vi "Lab Panel V4.83.vi"() -> ()   [LabVIEW 2013] (continued)
                n1247 = Equal?(x=w2130, y=2) -> (x = y?=w2133:bool)
                n1248 = local read "DISP LAB03-2"() -> (w2135:T4)
                n1249 = Unbundle(w2135) -> ("STATUS"=w2136:string)  [unwired: 2 out]
                n1250 = Equal?(x=w2136, y="RUN") -> (x = y?=w2132:bool)
                n1251 = And(x=w2132, y=w2133) -> (x .and. y?=w2131:bool)
                n1252 = case shown="True" w2131 {
                  tunnel: w2135 -> [_ w2139]
                  tunnel: w2129 -> [_ w2142]
                  frame False {
                  }
                  frame True {
                    n1253 = local read "SET LAB03-2"() -> (w2141:T5)
                    n1254 = local read "TDMS LAB03-2"() -> (w2138:refnum<k34>)
                    n1255 = Unbundle(w2139) -> ("CYCLE"=w2143:dbl)  [unwired: 2 out]
                    n1256 = Unbundle(w2141) -> ("T-RISE mins"=w2140:dbl)  [unwired: 4 out]
                    n1257 = Greater Or Equal?(x=w2143, y=w2142) -> (x >= y?=w2144:bool)
                    n1258 = case shown="True" w2144 {
                      tunnel: w2140 -> [w2147 _]
                      tunnel: w2139 -> [w2146 _]
                      tunnel: w2138 -> [w2145 _]
                      frame True {
                        n1259 = stacked-sequence {
                          tunnel: w2147 -> [w2150 _]
                          tunnel: w2146 -> [_ w2155]
                          tunnel: w2145 -> [w2148 _]
                          frame #0 {
                            n1260 = Build Array("T-RISE") -> (w2152:string[])
                            n1261 = Build Array(w2150) -> (w2151:dbl[])
                            n1262 = TDMS Write(0:w2148, 5:"TEST PASS", 7:w2152, 9:w2151) -> (15:w2154:errorcluster)  [unwired: 2 in, 3 out]
                            n1263 = local write "data file error"(w2154) -> ()
                          }
                          frame #1 {
                            n1264 = Bundle(cluster=w2155, "STATUS"="T-RISE PASS") -> (w2157:T4)  [unwired: 2 in]
                            n1265 = local write "RESULT LAB03-2"(TRUE) -> ()
                            n1266 = local write "DISP LAB03-2"(w2157) -> ()
                          }
                        }
                      }
                      frame False {
                      }
                    }
                  }
                }
              }
              frame #6 {
                # "LAB04-1"
                n1267 = Equal?(x=w2160, y=2) -> (x = y?=w2163:bool)
                n1268 = local read "DISP LAB04-1"() -> (w2165:T4)
                n1269 = Unbundle(w2165) -> ("STATUS"=w2166:string)  [unwired: 2 out]
                n1270 = Equal?(x=w2166, y="RUN") -> (x = y?=w2162:bool)
                n1271 = And(x=w2162, y=w2163) -> (x .and. y?=w2161:bool)
                n1272 = case shown="True" w2161 {
                  tunnel: w2165 -> [_ w2169]
                  tunnel: w2159 -> [_ w2172]
                  frame False {
                  }
                  frame True {
                    n1273 = local read "SET LAB04-1"() -> (w2171:T5)
                    n1274 = local read "TDMS LAB04-1"() -> (w2168:refnum<k34>)
                    n1275 = Unbundle(w2169) -> ("CYCLE"=w2173:dbl)  [unwired: 2 out]
                    n1276 = Unbundle(w2171) -> ("T-RISE mins"=w2170:dbl)  [unwired: 4 out]
                    n1277 = Greater Or Equal?(x=w2173, y=w2172) -> (x >= y?=w2174:bool)
                    n1278 = case shown="True" w2174 {
                      tunnel: w2170 -> [w2177 _]
                      tunnel: w2169 -> [w2176 _]
                      tunnel: w2168 -> [w2175 _]
                      frame True {
                        n1279 = stacked-sequence {
                          tunnel: w2177 -> [w2180 _]
                          tunnel: w2176 -> [_ w2185]
                          tunnel: w2175 -> [w2178 _]
                          frame #0 {
                            n1280 = Build Array("T-RISE") -> (w2182:string[])
                            n1281 = Build Array(w2180) -> (w2181:dbl[])
                            n1282 = TDMS Write(0:w2178, 5:"TEST PASS", 7:w2182, 9:w2181) -> (15:w2184:errorcluster)  [unwired: 2 in, 3 out]
                            n1283 = local write "data file error"(w2184) -> ()
                          }
                          frame #1 {
                            n1284 = Bundle(cluster=w2185, "STATUS"="T-RISE PASS") -> (w2187:T4)  [unwired: 2 in]
                            n1285 = local write "RESULT LAB04-1"(TRUE) -> ()
                            n1286 = local write "DISP LAB04-1"(w2187) -> ()
                          }
                        }
                      }
                      frame False {
                      }
                    }
                  }
                }
              }
              frame #7 {
                # "LAB04-2"
                n1287 = Equal?(x=w2190, y=2) -> (x = y?=w2193:bool)
                n1288 = local read "DISP LAB04-2"() -> (w2195:T4)
                n1289 = Unbundle(w2195) -> ("STATUS"=w2196:string)  [unwired: 2 out]
                n1290 = Equal?(x=w2196, y="RUN") -> (x = y?=w2192:bool)
                n1291 = And(x=w2192, y=w2193) -> (x .and. y?=w2191:bool)
                n1292 = case shown="True" w2191 {
                  tunnel: w2195 -> [_ w2199]
                  tunnel: w2189 -> [_ w2202]
                  frame False {
                  }
                  frame True {
                    n1293 = local read "SET LAB04-2"() -> (w2201:T5)
                    n1294 = local read "TDMS LAB04-2"() -> (w2198:refnum<k34>)
                    n1295 = Unbundle(w2199) -> ("CYCLE"=w2203:dbl)  [unwired: 2 out]
                    n1296 = Unbundle(w2201) -> ("T-RISE mins"=w2200:dbl)  [unwired: 4 out]
                    n1297 = Greater Or Equal?(x=w2203, y=w2202) -> (x >= y?=w2204:bool)
                    n1298 = case shown="True" w2204 {
                      tunnel: w2200 -> [w2207 _]
                      tunnel: w2199 -> [w2206 _]
                      tunnel: w2198 -> [w2205 _]
                      frame True {
                        n1299 = stacked-sequence {
                          tunnel: w2207 -> [w2210 _]
                          tunnel: w2206 -> [_ w2215]
                          tunnel: w2205 -> [w2208 _]
                          frame #0 {
                            n1300 = Build Array("T-RISE") -> (w2212:string[])
                            n1301 = Build Array(w2210) -> (w2211:dbl[])
                            n1302 = TDMS Write(0:w2208, 5:"TEST PASS", 7:w2212, 9:w2211) -> (15:w2214:errorcluster)  [unwired: 2 in, 3 out]
                            n1303 = local write "data file error"(w2214) -> ()
                          }
                          frame #1 {
                            n1304 = Bundle(cluster=w2215, "STATUS"="T-RISE PASS") -> (w2217:T4)  [unwired: 2 in]
                            n1305 = local write "RESULT LAB04-2"(TRUE) -> ()
                            n1306 = local write "DISP LAB04-2"(w2217) -> ()
                          }
                        }
                      }
                      frame False {
                      }
                    }
                  }
                }
              }
              frame #8 {
                # "LAB05-1"
                n1307 = Equal?(x=w2220, y=2) -> (x = y?=w2223:bool)
                n1308 = local read "DISP LAB05-1"() -> (w2225:T4)
                n1309 = Unbundle(w2225) -> ("STATUS"=w2226:string)  [unwired: 2 out]
                n1310 = Equal?(x=w2226, y="RUN") -> (x = y?=w2222:bool)
                n1311 = And(x=w2222, y=w2223) -> (x .and. y?=w2221:bool)
                n1312 = case shown="True" w2221 {
                  tunnel: w2225 -> [_ w2229]
                  tunnel: w2219 -> [_ w2232]
                  frame False {
                  }
                  frame True {
                    n1313 = local read "SET LAB05-1"() -> (w2231:T5)
                    n1314 = local read "TDMS LAB05-1"() -> (w2228:refnum<k34>)
                    n1315 = Unbundle(w2229) -> ("CYCLE"=w2233:dbl)  [unwired: 2 out]
                    n1316 = Unbundle(w2231) -> ("T-RISE mins"=w2230:dbl)  [unwired: 4 out]
                    n1317 = Greater Or Equal?(x=w2233, y=w2232) -> (x >= y?=w2234:bool)
                    n1318 = case shown="True" w2234 {
                      tunnel: w2230 -> [w2237 _]
                      tunnel: w2229 -> [w2236 _]
                      tunnel: w2228 -> [w2235 _]
                      frame True {
                        n1319 = stacked-sequence {
                          tunnel: w2237 -> [w2240 _]
                          tunnel: w2236 -> [_ w2245]
                          tunnel: w2235 -> [w2238 _]
                          frame #0 {
                            n1320 = Build Array("T-RISE") -> (w2242:string[])
                            n1321 = Build Array(w2240) -> (w2241:dbl[])
                            n1322 = TDMS Write(0:w2238, 5:"TEST PASS", 7:w2242, 9:w2241) -> (15:w2244:errorcluster)  [unwired: 2 in, 3 out]
                            n1323 = local write "data file error"(w2244) -> ()
                          }
                          frame #1 {
                            n1324 = Bundle(cluster=w2245, "STATUS"="T-RISE PASS") -> (w2247:T4)  [unwired: 2 in]
                            n1325 = local write "RESULT LAB05-1"(TRUE) -> ()
                            n1326 = local write "DISP LAB05-1"(w2247) -> ()
                          }
                        }
                      }
                      frame False {
                      }
                    }
                  }
                }
              }
              frame #9 {
                # "LAB05-2"
                n1327 = Equal?(x=w2250, y=2) -> (x = y?=w2253:bool)
                n1328 = local read "DISP LAB05-2"() -> (w2255:T4)
                n1329 = Unbundle(w2255) -> ("STATUS"=w2256:string)  [unwired: 2 out]
                n1330 = Equal?(x=w2256, y="RUN") -> (x = y?=w2252:bool)
                n1331 = And(x=w2252, y=w2253) -> (x .and. y?=w2251:bool)
                n1332 = case shown="True" w2251 {
                  tunnel: w2255 -> [_ w2259]
                  tunnel: w2249 -> [_ w2262]
                  frame False {
                  }
                  frame True {
                    n1333 = local read "SET LAB05-2"() -> (w2261:T5)
                    n1334 = local read "TDMS LAB05-2"() -> (w2258:refnum<k34>)
                    n1335 = Unbundle(w2259) -> ("CYCLE"=w2263:dbl)  [unwired: 2 out]
                    n1336 = Unbundle(w2261) -> ("T-RISE mins"=w2260:dbl)  [unwired: 4 out]
                    n1337 = Greater Or Equal?(x=w2263, y=w2262) -> (x >= y?=w2264:bool)
                    n1338 = case shown="True" w2264 {
                      tunnel: w2260 -> [w2267 _]
                      tunnel: w2259 -> [w2266 _]
                      tunnel: w2258 -> [w2265 _]
                      frame True {
                        n1339 = stacked-sequence {
                          tunnel: w2267 -> [w2270 _]
                          tunnel: w2266 -> [_ w2275]
                          tunnel: w2265 -> [w2268 _]
                          frame #0 {
                            n1340 = Build Array("T-RISE") -> (w2272:string[])
                            n1341 = Build Array(w2270) -> (w2271:dbl[])
                            n1342 = TDMS Write(0:w2268, 5:"TEST PASS", 7:w2272, 9:w2271) -> (15:w2274:errorcluster)  [unwired: 2 in, 3 out]
                            n1343 = local write "data file error"(w2274) -> ()
                          }
                          frame #1 {
                            n1344 = Bundle(cluster=w2275, "STATUS"="T-RISE PASS") -> (w2277:T4)  [unwired: 2 in]
                            n1345 = local write "RESULT LAB05-2"(TRUE) -> ()
                            n1346 = local write "DISP LAB05-2"(w2277) -> ()
                          }
                        }
                      }
                      frame False {
                      }
                    }
                  }
                }
              }
            }
          }
          frame #6 {
            # "end test & close test files"
            n1347 = stacked-sequence {
              tunnel: w2288 -> [_ _ _ _ _ _ _ _ _ _]
              tunnel: w2289 -> [_ _ _ _ _ _ _ _ _ _]
              tunnel: w2287 -> [_ _ _ _ _ _ _ _ _ _]
              tunnel: w2286 -> [_ _ _ _ _ _ _ _ _ _]
              tunnel: w2285 -> [_ _ _ _ _ _ _ _ _ _]
              tunnel: w2284 -> [_ _ _ _ _ _ _ _ _ _]
              tunnel: w2283 -> [_ _ _ _ _ _ _ _ _ _]
              tunnel: w2282 -> [_ _ _ _ _ _ _ _ _ _]
              tunnel: w2281 -> [_ _ _ _ _ _ _ _ _ _]
              tunnel: w2280 -> [_ _ _ _ _ _ _ _ _ _]
              frame #0 {
                # "LAB01-1"
                n1348 = local read "DISP LAB01-1"() -> (w2293:T4)
                n1349 = local read "run lab01-1"() -> (w2290:bool)
                n1350 = local read "TDMS LAB01-1"() -> (w2291:refnum<k34>)
                n1351 = Unbundle(w2293) -> ("CYCLE"=w2294:dbl, "STATUS"=w2292:string)  [unwired: 1 out]
                n1352 = case shown="True" w2290 {
                  tunnel: w2294 -> [_ w2298]
                  tunnel: w2293 -> [_ w2297]
                  tunnel: w2292 -> [_ w2296]
                  tunnel: w2291 -> [_ w2295]
                  frame False {
                  }
                  frame True {
                    n1353 = Not Equal?(x=w2296, y="RUN") -> (x != y?=w2299:bool)
                    n1354 = Greater?(x=w2298, y=2.0) -> (0:w2301:bool)
                    n1355 = And(x=w2301, y=w2299) -> (x .and. y?=w2300:bool)
                    n1356 = case shown="True" w2300 {
                      tunnel: w2297 -> [_ w2305]
                      tunnel: w2295 -> [_ w2304]
                      frame False {
                      }
                      frame True {
                        n1357 = stacked-sequence {
                          tunnel: w2305 -> [w2309 _ _]
                          tunnel: w2304 -> [_ w2311 _]
                          frame #0 {
                            w2306 = FALSE
                            n1358 = local write "mail control"("END") -> ()
                            n1359 = Bundle(cluster=w2309) -> (w2308:T4)  [unwired: 3 in]
                            n1360 = local write "DISP LAB01-1"(w2308) -> ()
                            n1361 = local write "O/I  LAB01-1"(w2306) -> ()
                            n1362 = local write "run lab01-1"(w2306) -> ()
                            n1363 = local write "RUN LAB01-1"(w2306) -> ()
                          }
                          frame #1 {
                            n1364 = TDMS Close(11:w2311) -> (0:w2310:errorcluster)  [unwired: 1 in, 1 out]
                            n1365 = local write "data file error"(w2310) -> ()
                          }
                          frame #2 {
                            n1366 = stacked-sequence {
                              tunnel: "LAB01-1" -> [w2314 w2316]
                              frame #0 {
                                n1367 = call "sub vi - defrag tdms v1.vi"("panel id"=w2314) -> ("error out"=w2313:errorcluster)  [unwired: 10 in]
                                n1368 = local write "data file error"(w2313) -> ()
                              }
                              frame #1 {
                                n1369 = call "Save data file to network drive v1.vi"("panel id"=w2316) -> ("network file save error"=w2315:errorcluster)  [unwired: 9 in, 1 out]
                                n1370 = local write "data file error"(w2315) -> ()
                              }
                            }
                          }
                        }
                      }
                    }
                  }
                }
              }
              frame #1 {
                # "LAB01-2"
                n1371 = local read "run lab01-2"() -> (w2317:bool)
                n1372 = case shown="True" w2317 {
                  frame False {
                  }
                  frame True {
                    n1373 = local read "DISP LAB01-2"() -> (w2324:T4)
                    n1374 = local read "TDMS LAB01-2"() -> (w2323:refnum<k34>)
                    n1375 = Unbundle(w2324) -> ("CYCLE"=w2320:dbl, "STATUS"=w2325:string)  [unwired: 1 out]
                    n1376 = Not Equal?(x=w2325, y="RUN") -> (x != y?=w2319:bool)
                    n1377 = Greater?(x=w2320, y=2.0) -> (0:w2321:bool)
                    n1378 = And(x=w2321, y=w2319) -> (x .and. y?=w2318:bool)
                    n1379 = case shown="True" w2318 {
                      tunnel: w2324 -> [_ w2328]
                      tunnel: w2323 -> [_ w2327]
                      frame False {
                      }
                      frame True {
                        n1380 = stacked-sequence {
                          tunnel: w2328 -> [w2331 _ _]
                          tunnel: w2327 -> [_ w2333 _]
                          frame #0 {
                            w2329 = FALSE
                            n1381 = local write "mail control"("END") -> ()
                            n1382 = Bundle(cluster=w2331) -> (w2332:T4)  [unwired: 3 in]
                            n1383 = local write "RUN LAB01-2"(w2329) -> ()
                            n1384 = local write "run lab01-2"(w2329) -> ()
                            n1385 = local write "O/I  LAB01-2"(w2329) -> ()
                            n1386 = local write "DISP LAB01-2"(w2332) -> ()
                          }
                          frame #1 {
                            n1387 = TDMS Close(11:w2333) -> (0:w2334:errorcluster)  [unwired: 1 in, 1 out]
                            n1388 = local write "data file error"(w2334) -> ()
                          }
                          frame #2 {
                            n1389 = stacked-sequence {
                              tunnel: "LAB01-2" -> [w2337 w2339]
                              frame #0 {
                                n1390 = call "sub vi - defrag tdms v1.vi"("panel id"=w2337) -> ("error out"=w2336:errorcluster)  [unwired: 10 in]
                                n1391 = local write "data file error"(w2336) -> ()
                              }
                              frame #1 {
                                n1392 = call "Save data file to network drive v1.vi"("panel id"=w2339) -> ("network file save error"=w2338:errorcluster)  [unwired: 9 in, 1 out]
                                n1393 = local write "data file error"(w2338) -> ()
                              }
                            }
                          }
                        }
                      }
                    }
                  }
                }
              }
              frame #2 {
                # "LAB02-1"
                n1394 = local read "run lab02-1"() -> (w2340:bool)
                n1395 = case shown="True" w2340 {
                  frame False {
                  }
                  frame True {
                    n1396 = local read "DISP LAB02-1"() -> (w2347:T4)
                    n1397 = Unbundle(w2347) -> ("CYCLE"=w2343:dbl, "STATUS"=w2348:string)  [unwired: 1 out]
                    n1398 = local read "TDMS LAB02-1"() -> (w2346:refnum<k34>)
                    n1399 = Not Equal?(x=w2348, y="RUN") -> (x != y?=w2342:bool)
                    n1400 = Greater?(x=w2343, y=2.0) -> (0:w2344:bool)
                    n1401 = And(x=w2344, y=w2342) -> (x .and. y?=w2341:bool)
                    n1402 = case shown="True" w2341 {
                      tunnel: w2347 -> [_ w2351]
                      tunnel: w2346 -> [_ w2350]
                      frame False {
                      }
                      frame True {
                        n1403 = stacked-sequence {
                          tunnel: w2351 -> [w2354 _ _]
                          tunnel: w2350 -> [_ w2356 _]
                          frame #0 {
                            w2352 = FALSE
                            n1404 = local write "mail control"("END") -> ()
                            n1405 = Bundle(cluster=w2354) -> (w2355:T4)  [unwired: 3 in]
                            n1406 = local write "O/I  LAB02-1"(w2352) -> ()
                            n1407 = local write "RUN LAB02-1"(w2352) -> ()
                            n1408 = local write "run lab02-1"(w2352) -> ()
                            n1409 = local write "DISP LAB02-1"(w2355) -> ()
                          }
                          frame #1 {
                            n1410 = TDMS Close(11:w2356) -> (0:w2357:errorcluster)  [unwired: 1 in, 1 out]
                            n1411 = local write "data file error"(w2357) -> ()
                          }
                          frame #2 {
                            n1412 = stacked-sequence {
                              tunnel: "LAB02-1" -> [w2360 w2362]
                              frame #0 {
                                n1413 = call "sub vi - defrag tdms v1.vi"("panel id"=w2360) -> ("error out"=w2359:errorcluster)  [unwired: 10 in]
                                n1414 = local write "data file error"(w2359) -> ()
                              }
                              frame #1 {
                                n1415 = call "Save data file to network drive v1.vi"("panel id"=w2362) -> ("network file save error"=w2361:errorcluster)  [unwired: 9 in, 1 out]
                                n1416 = local write "data file error"(w2361) -> ()
                              }
                            }
                          }
                        }
                      }
                    }
                  }
                }
              }
              frame #3 {
                # "LAB02-2"
                n1417 = local read "run lab02-2"() -> (w2363:bool)
                n1418 = case shown="True" w2363 {
                  frame False {
                  }
                  frame True {
                    n1419 = local read "DISP LAB02-2"() -> (w2370:T4)
                    n1420 = local read "TDMS LAB02-2"() -> (w2369:refnum<k34>)
                    n1421 = Unbundle(w2370) -> ("CYCLE"=w2366:dbl, "STATUS"=w2371:string)  [unwired: 1 out]
                    n1422 = Not Equal?(x=w2371, y="RUN") -> (x != y?=w2365:bool)
                    n1423 = Greater?(x=w2366, y=2.0) -> (0:w2367:bool)
                    n1424 = And(x=w2367, y=w2365) -> (x .and. y?=w2364:bool)
                    n1425 = case shown="True" w2364 {
                      tunnel: w2370 -> [_ w2374]
                      tunnel: w2369 -> [_ w2373]
                      frame False {
                      }
                      frame True {
                        n1426 = stacked-sequence {
                          tunnel: w2374 -> [w2377 _ _]
                          tunnel: w2373 -> [_ w2379 _]
                          frame #0 {
                            w2375 = FALSE
                            n1427 = local write "mail control"("END") -> ()
                            n1428 = Bundle(cluster=w2377) -> (w2378:T4)  [unwired: 3 in]
                            n1429 = local write "O/I  LAB02-2"(w2375) -> ()
                            n1430 = local write "run lab02-2"(w2375) -> ()
                            n1431 = local write "RUN LAB02-2"(w2375) -> ()
                            n1432 = local write "DISP LAB02-2"(w2378) -> ()
                          }
                          frame #1 {
                            n1433 = TDMS Close(11:w2379) -> (0:w2380:errorcluster)  [unwired: 1 in, 1 out]
                            n1434 = local write "data file error"(w2380) -> ()
                          }
                          frame #2 {
                            n1435 = stacked-sequence {
                              tunnel: "LAB02-2" -> [w2383 w2385]
                              frame #0 {
                                n1436 = call "sub vi - defrag tdms v1.vi"("panel id"=w2383) -> ("error out"=w2382:errorcluster)  [unwired: 10 in]
                                n1437 = local write "data file error"(w2382) -> ()
                              }
                              frame #1 {
                                n1438 = call "Save data file to network drive v1.vi"("panel id"=w2385) -> ("network file save error"=w2384:errorcluster)  [unwired: 9 in, 1 out]
                                n1439 = local write "data file error"(w2384) -> ()
                              }
                            }
                          }
                        }
                      }
                    }
                  }
                }
              }
              frame #4 {
                # "LAB03-1"
                n1440 = local read "run lab03-1"() -> (w2386:bool)
                n1441 = case shown="True" w2386 {
                  frame False {
                  }
                  frame True {
                    n1442 = local read "DISP LAB03-1"() -> (w2393:T4)
                    n1443 = local read "TDMS LAB03-1"() -> (w2392:refnum<k34>)
                    n1444 = Unbundle(w2393) -> ("CYCLE"=w2389:dbl, "STATUS"=w2394:string)  [unwired: 1 out]
                    n1445 = Not Equal?(x=w2394, y="RUN") -> (x != y?=w2388:bool)
                    n1446 = Greater?(x=w2389, y=2.0) -> (0:w2390:bool)
                    n1447 = And(x=w2390, y=w2388) -> (x .and. y?=w2387:bool)
                    n1448 = case shown="True" w2387 {
                      tunnel: w2393 -> [_ w2397]
                      tunnel: w2392 -> [_ w2396]
                      frame False {
                      }
                      frame True {
                        n1449 = stacked-sequence {
                          tunnel: w2397 -> [w2400 _ _]
                          tunnel: w2396 -> [_ w2402 _]
                          frame #0 {
                            w2398 = FALSE
                            n1450 = local write "mail control"("END") -> ()
                            n1451 = Bundle(cluster=w2400) -> (w2401:T4)  [unwired: 3 in]
                            n1452 = local write "O/I  LAB03-1"(w2398) -> ()
                            n1453 = local write "run lab03-1"(w2398) -> ()
                            n1454 = local write "RUN LAB03-1"(w2398) -> ()
                            n1455 = local write "DISP LAB03-1"(w2401) -> ()
                          }
                          frame #1 {
                            n1456 = TDMS Close(11:w2402) -> (0:w2403:errorcluster)  [unwired: 1 in, 1 out]
                            n1457 = local write "data file error"(w2403) -> ()
                          }
                          frame #2 {
                            n1458 = stacked-sequence {
                              tunnel: "LAB03-1" -> [w2406 w2408]
                              frame #0 {
                                n1459 = call "sub vi - defrag tdms v1.vi"("panel id"=w2406) -> ("error out"=w2405:errorcluster)  [unwired: 10 in]
                                n1460 = local write "data file error"(w2405) -> ()
                              }
                              frame #1 {
                                n1461 = call "Save data file to network drive v1.vi"("panel id"=w2408) -> ("network file save error"=w2407:errorcluster)  [unwired: 9 in, 1 out]
                                n1462 = local write "data file error"(w2407) -> ()
                              }
                            }
                          }
                        }
                      }
                    }
                  }
                }
              }
              frame #5 {
                # "LAB03-2"
                n1463 = local read "run lab03-2"() -> (w2409:bool)
                n1464 = case shown="True" w2409 {
                  frame False {
                  }
                  frame True {
                    n1465 = local read "DISP LAB03-2"() -> (w2416:T4)
                    n1466 = Unbundle(w2416) -> ("CYCLE"=w2412:dbl, "STATUS"=w2417:string)  [unwired: 1 out]
                    n1467 = local read "TDMS LAB03-2"() -> (w2415:refnum<k34>)
                    n1468 = Not Equal?(x=w2417, y="RUN") -> (x != y?=w2411:bool)
                    n1469 = Greater?(x=w2412, y=2.0) -> (0:w2413:bool)
                    n1470 = And(x=w2413, y=w2411) -> (x .and. y?=w2410:bool)
                    n1471 = case shown="True" w2410 {
                      tunnel: w2416 -> [_ w2420]
                      tunnel: w2415 -> [_ w2419]
                      frame False {
                      }
                      frame True {
                        n1472 = stacked-sequence {
                          tunnel: w2420 -> [w2423 _ _]
                          tunnel: w2419 -> [_ w2425 _]
                          frame #0 {
                            w2421 = FALSE
                            n1473 = local write "mail control"("END") -> ()
                            n1474 = Bundle(cluster=w2423) -> (w2424:T4)  [unwired: 3 in]
                            n1475 = local write "RUN LAB03-2"(w2421) -> ()
                            n1476 = local write "O/I  LAB03-2"(w2421) -> ()
                            n1477 = local write "DISP LAB03-2"(w2424) -> ()
                            n1478 = local write "run lab03-2"(w2421) -> ()
                          }
                          frame #1 {
                            n1479 = TDMS Close(11:w2425) -> (0:w2426:errorcluster)  [unwired: 1 in, 1 out]
                            n1480 = local write "data file error"(w2426) -> ()
                          }
                          frame #2 {
                            n1481 = stacked-sequence {
                              tunnel: "LAB03-2" -> [w2429 w2431]
                              frame #0 {
                                n1482 = call "sub vi - defrag tdms v1.vi"("panel id"=w2429) -> ("error out"=w2428:errorcluster)  [unwired: 10 in]
                                n1483 = local write "data file error"(w2428) -> ()
                              }
                              frame #1 {
                                n1484 = call "Save data file to network drive v1.vi"("panel id"=w2431) -> ("network file save error"=w2430:errorcluster)  [unwired: 9 in, 1 out]
                                n1485 = local write "data file error"(w2430) -> ()
                              }
                            }
                          }
                        }
                      }
                    }
                  }
                }
              }
              frame #6 {
                # "LAB04-1"
                n1486 = local read "run lab04-1"() -> (w2432:bool)
                n1487 = case shown="True" w2432 {
                  frame False {
                  }
                  frame True {
                    n1488 = local read "DISP LAB04-1"() -> (w2439:T4)
                    n1489 = Unbundle(w2439) -> ("CYCLE"=w2435:dbl, "STATUS"=w2440:string)  [unwired: 1 out]
                    n1490 = local read "TDMS LAB04-1"() -> (w2438:refnum<k34>)
                    n1491 = Not Equal?(x=w2440, y="RUN") -> (x != y?=w2434:bool)
                    n1492 = Greater?(x=w2435, y=2.0) -> (0:w2436:bool)
                    n1493 = And(x=w2436, y=w2434) -> (x .and. y?=w2433:bool)
                    n1494 = case shown="True" w2433 {
                      tunnel: w2439 -> [_ w2443]
                      tunnel: w2438 -> [_ w2442]
                      frame False {
                      }
                      frame True {
                        n1495 = stacked-sequence {
                          tunnel: w2443 -> [w2446 _ _]
                          tunnel: w2442 -> [_ w2448 _]
                          frame #0 {
                            w2444 = FALSE
                            n1496 = local write "mail control"("END") -> ()
                            n1497 = Bundle(cluster=w2446) -> (w2447:T4)  [unwired: 3 in]
                            n1498 = local write "RUN LAB04-1"(w2444) -> ()
                            n1499 = local write "O/I  LAB04-1"(w2444) -> ()
                            n1500 = local write "run lab04-1"(w2444) -> ()
                            n1501 = local write "DISP LAB04-1"(w2447) -> ()
                          }
                          frame #1 {
                            n1502 = TDMS Close(11:w2448) -> (0:w2449:errorcluster)  [unwired: 1 in, 1 out]
                            n1503 = local write "data file error"(w2449) -> ()
                          }
                          frame #2 {
                            n1504 = stacked-sequence {
                              tunnel: "LAB04-1" -> [w2452 w2454]
                              frame #0 {
                                n1505 = call "sub vi - defrag tdms v1.vi"("panel id"=w2452) -> ("error out"=w2451:errorcluster)  [unwired: 10 in]
                                n1506 = local write "data file error"(w2451) -> ()
                              }
                              frame #1 {
                                n1507 = call "Save data file to network drive v1.vi"("panel id"=w2454) -> ("network file save error"=w2453:errorcluster)  [unwired: 9 in, 1 out]
                                n1508 = local write "data file error"(w2453) -> ()
                              }
                            }
                          }
                        }
                      }
                    }
                  }
                }
              }
              frame #7 {
                # "LAB04-2"
                n1509 = local read "run lab04-2"() -> (w2455:bool)
                n1510 = case shown="True" w2455 {
                  frame False {
                  }
                  frame True {
                    n1511 = local read "DISP LAB04-2"() -> (w2462:T4)
                    n1512 = Unbundle(w2462) -> ("CYCLE"=w2458:dbl, "STATUS"=w2463:string)  [unwired: 1 out]
                    n1513 = Not Equal?(x=w2463, y="RUN") -> (x != y?=w2457:bool)
                    n1514 = local read "TDMS LAB04-2"() -> (w2461:refnum<k34>)
                    n1515 = Greater?(x=w2458, y=2.0) -> (0:w2459:bool)
                    n1516 = And(x=w2459, y=w2457) -> (x .and. y?=w2456:bool)
                    n1517 = case shown="True" w2456 {
                      tunnel: w2462 -> [_ w2466]
                      tunnel: w2461 -> [_ w2465]
                      frame False {
                      }
                      frame True {
                        n1518 = stacked-sequence {
                          tunnel: w2466 -> [w2469 _ _]
                          tunnel: w2465 -> [_ w2471 _]
                          frame #0 {
                            w2467 = FALSE
                            n1519 = local write "mail control"("END") -> ()
                            n1520 = Bundle(cluster=w2469) -> (w2470:T4)  [unwired: 3 in]
                            n1521 = local write "O/I  LAB04-2"(w2467) -> ()
                            n1522 = local write "RUN LAB04-2"(w2467) -> ()
                            n1523 = local write "run lab04-2"(w2467) -> ()
                            n1524 = local write "DISP LAB04-2"(w2470) -> ()
                          }
                          frame #1 {
                            n1525 = TDMS Close(11:w2471) -> (0:w2472:errorcluster)  [unwired: 1 in, 1 out]
                            n1526 = local write "data file error"(w2472) -> ()
                          }
                          frame #2 {
                            n1527 = stacked-sequence {
                              tunnel: "LAB04-2" -> [w2475 w2477]
                              frame #0 {
                                n1528 = call "sub vi - defrag tdms v1.vi"("panel id"=w2475) -> ("error out"=w2474:errorcluster)  [unwired: 10 in]
                                n1529 = local write "data file error"(w2474) -> ()
                              }
                              frame #1 {
                                n1530 = call "Save data file to network drive v1.vi"("panel id"=w2477) -> ("network file save error"=w2476:errorcluster)  [unwired: 9 in, 1 out]
                                n1531 = local write "data file error"(w2476) -> ()
                              }
                            }
                          }
                        }
                      }
                    }
                  }
                }
              }
              frame #8 {
                # "LAB05-1"
                n1532 = local read "run lab05-1"() -> (w2478:bool)
                n1533 = case shown="True" w2478 {
                  frame False {
                  }
                  frame True {
                    n1534 = local read "DISP LAB05-1"() -> (w2485:T4)
                    n1535 = Unbundle(w2485) -> ("CYCLE"=w2481:dbl, "STATUS"=w2486:string)  [unwired: 1 out]
                    n1536 = Not Equal?(x=w2486, y="RUN") -> (x != y?=w2480:bool)
                    n1537 = local read "TDMS LAB05-1"() -> (w2484:refnum<k34>)
                    n1538 = Greater?(x=w2481, y=2.0) -> (0:w2482:bool)
                    n1539 = And(x=w2482, y=w2480) -> (x .and. y?=w2479:bool)
                    n1540 = case shown="True" w2479 {
                      tunnel: w2485 -> [_ w2489]
                      tunnel: w2484 -> [_ w2488]
                      frame False {
                      }
                      frame True {
                        n1541 = stacked-sequence {
                          tunnel: w2489 -> [w2492 _ _]
                          tunnel: w2488 -> [_ w2494 _]
                          frame #0 {
                            w2490 = FALSE
                            n1542 = local write "mail control"("END") -> ()
                            n1543 = Bundle(cluster=w2492) -> (w2493:T4)  [unwired: 3 in]
                            n1544 = local write "O/I  LAB05-1"(w2490) -> ()
                            n1545 = local write "RUN LAB05-1"(w2490) -> ()
                            n1546 = local write "run lab05-1"(w2490) -> ()
                            n1547 = local write "DISP LAB05-1"(w2493) -> ()
                          }
                          frame #1 {
                            n1548 = TDMS Close(11:w2494) -> (0:w2495:errorcluster)  [unwired: 1 in, 1 out]
                            n1549 = local write "data file error"(w2495) -> ()
                          }
                          frame #2 {
                            n1550 = stacked-sequence {
                              tunnel: "LAB05-1" -> [w2498 w2500]
                              frame #0 {
                                n1551 = call "sub vi - defrag tdms v1.vi"("panel id"=w2498) -> ("error out"=w2497:errorcluster)  [unwired: 10 in]
                                n1552 = local write "data file error"(w2497) -> ()
                              }
                              frame #1 {
                                n1553 = call "Save data file to network drive v1.vi"("panel id"=w2500) -> ("network file save error"=w2499:errorcluster)  [unwired: 9 in, 1 out]
                                n1554 = local write "data file error"(w2499) -> ()
                              }
                            }
                          }
                        }
                      }
                    }
                  }
                }
              }
              frame #9 {
                # "LAB05-2"
                n1555 = local read "run lab05-2"() -> (w2501:bool)
                n1556 = case shown="True" w2501 {
                  frame False {
                  }
                  frame True {
                    n1557 = local read "DISP LAB05-2"() -> (w2508:T4)
                    n1558 = Unbundle(w2508) -> ("CYCLE"=w2504:dbl, "STATUS"=w2509:string)  [unwired: 1 out]
                    n1559 = Not Equal?(x=w2509, y="RUN") -> (x != y?=w2503:bool)
                    n1560 = local read "TDMS LAB05-2"() -> (w2507:refnum<k34>)
                    n1561 = Greater?(x=w2504, y=2.0) -> (0:w2505:bool)
                    n1562 = And(x=w2505, y=w2503) -> (x .and. y?=w2502:bool)
                    n1563 = case shown="True" w2502 {
                      tunnel: w2508 -> [_ w2512]
                      tunnel: w2507 -> [_ w2511]
                      frame False {
                      }
                      frame True {
                        n1564 = stacked-sequence {
                          tunnel: w2512 -> [w2515 _ _]
                          tunnel: w2511 -> [_ w2517 _]
                          frame #0 {
                            w2513 = FALSE
                            n1565 = local write "mail control"("END") -> ()
                            n1566 = Bundle(cluster=w2515) -> (w2516:T4)  [unwired: 3 in]
                            n1567 = local write "RUN LAB05-2"(w2513) -> ()
                            n1568 = local write "O/I  LAB05-2"(w2513) -> ()
                            n1569 = local write "run lab05-2"(w2513) -> ()
                            n1570 = local write "DISP LAB05-2"(w2516) -> ()
                          }
                          frame #1 {
                            n1571 = TDMS Close(11:w2517) -> (0:w2518:errorcluster)  [unwired: 1 in, 1 out]
                            n1572 = local write "data file error"(w2518) -> ()
                          }
                          frame #2 {
                            n1573 = stacked-sequence {
                              tunnel: "LAB05-2" -> [w2521 w2523]
                              frame #0 {
                                n1574 = call "sub vi - defrag tdms v1.vi"("panel id"=w2521) -> ("error out"=w2520:errorcluster)  [unwired: 10 in]
                                n1575 = local write "data file error"(w2520) -> ()
                              }
                              frame #1 {
                                n1576 = call "Save data file to network drive v1.vi"("panel id"=w2523) -> ("network file save error"=w2522:errorcluster)  [unwired: 9 in, 1 out]
                                n1577 = local write "data file error"(w2522) -> ()
                              }
                            }
                          }
                        }
                      }
                    }
                  }
                }
              }
            }
            n1578 = local read "Network Directory"() -> (w2279:path)
            n1579 = global write "Global 1.vi" "Network Drive"(w2279) -> ()
          }
          frame #7 {
            # "disable functions"
            n1580 = stacked-sequence {
              tunnel: w2533 -> [w2547 _ w2603]
              tunnel: w2532 -> [w2542 _ w2602]
              tunnel: w2531 -> [w2541 _ w2601]
              tunnel: w2530 -> [w2539 _ w2600]
              tunnel: w2529 -> [w2540 _ w2599]
              tunnel: w2528 -> [_ w2564 w2598]
              tunnel: w2527 -> [_ w2565 w2597]
              tunnel: w2526 -> [_ w2566 w2596]
              tunnel: w2525 -> [_ w2567 w2595]
              tunnel: w2524 -> [_ w2568 w2594]
              frame #0 {
                n1581 = Select(t=2, s=w2539, f=0) -> (s? t:f=w2535:i32)
                n1582 = Select(t=2, s=w2541, f=0) -> (s? t:f=w2536:i32)
                n1583 = Select(t=2, s=w2540, f=0) -> (s? t:f=w2534:i32)
                n1584 = Select(t=2, s=w2547, f=0) -> (s? t:f=w2538:i32)
                n1585 = Select(t=2, s=w2542, f=0) -> (s? t:f=w2537:i32)
                n1586 = property on="SELECT LAB02-2" class="RadioBtnsControl (strict)"("DisabledEnum"=w2535) -> ()  [unwired: 2 in, 2 out]
                n1587 = property on="SELECT LAB02-1" class="RadioBtnsControl (strict)"("DisabledEnum"=w2536) -> ()  [unwired: 2 in, 2 out]
                n1588 = property on="SELECT LAB03-1" class="RadioBtnsControl (strict)"("DisabledEnum"=w2534) -> ()  [unwired: 2 in, 2 out]
                n1589 = property on="SELECT LAB01-1" class="RadioBtnsControl (strict)"("DisabledEnum"=w2538) -> ()  [unwired: 2 in, 2 out]
                n1590 = property on="SELECT LAB01-2" class="RadioBtnsControl (strict)"("DisabledEnum"=w2537) -> ()  [unwired: 2 in, 2 out]
                n1591 = Not(x=w2547) -> (.not. x?=w2548:bool)
                n1592 = property on="RESULT LAB01-1" class="Bool (strict)"("Visible"=w2548) -> ()  [unwired: 2 in, 2 out]
                n1593 = Not(x=w2542) -> (.not. x?=w2546:bool)
                n1594 = Not(x=w2541) -> (.not. x?=w2545:bool)
                n1595 = Not(x=w2539) -> (.not. x?=w2544:bool)
                n1596 = property on="RESULT LAB01-2" class="Bool (strict)"("Visible"=w2546) -> ()  [unwired: 2 in, 2 out]
                n1597 = Not(x=w2540) -> (.not. x?=w2543:bool)
                n1598 = property on="RESULT LAB02-1" class="Bool (strict)"("Visible"=w2545) -> ()  [unwired: 2 in, 2 out]
                n1599 = property on="RESULT LAB02-2" class="Bool (strict)"("Visible"=w2544) -> ()  [unwired: 2 in, 2 out]
                n1600 = property on="RESULT LAB03-1" class="Bool (strict)"("Visible"=w2543) -> ()  [unwired: 2 in, 2 out]
                n1601 = property on="SET LAB01-1" class="Clust (strict)"("DisabledEnum"=w2538) -> ()  [unwired: 2 in, 2 out]
                n1602 = property on="SET LAB01-2" class="Clust (strict)"("DisabledEnum"=w2537) -> ()  [unwired: 2 in, 2 out]
                n1603 = property on="SET LAB02-1" class="Clust (strict)"("DisabledEnum"=w2536) -> ()  [unwired: 2 in, 2 out]
                n1604 = property on="SET LAB02-2" class="Clust (strict)"("DisabledEnum"=w2535) -> ()  [unwired: 2 in, 2 out]
                n1605 = property on="SET LAB03-1" class="Clust (strict)"("DisabledEnum"=w2534) -> ()  [unwired: 2 in, 2 out]
                n1606 = property on="O/I  LAB01-1" class="Bool (strict)"("DisabledEnum"=w2538) -> ()  [unwired: 2 in, 2 out]
                n1607 = property on="O/I  LAB01-2" class="Bool (strict)"("DisabledEnum"=w2537) -> ()  [unwired: 2 in, 2 out]
                n1608 = property on="O/I  LAB02-1" class="Bool (strict)"("DisabledEnum"=w2536) -> ()  [unwired: 2 in, 2 out]
                n1609 = property on="O/I  LAB02-2" class="Bool (strict)"("DisabledEnum"=w2535) -> ()  [unwired: 2 in, 2 out]
                n1610 = property on="O/I  LAB03-1" class="Bool (strict)"("DisabledEnum"=w2534) -> ()  [unwired: 2 in, 2 out]
              }
              frame #1 {
                n1611 = Select(t=2, s=w2568, f=0) -> (s? t:f=w2559:i32)
                n1612 = Select(t=2, s=w2567, f=0) -> (s? t:f=w2560:i32)
                n1613 = Select(t=2, s=w2564, f=0) -> (s? t:f=w2563:i32)
                n1614 = Select(t=2, s=w2565, f=0) -> (s? t:f=w2562:i32)
                n1615 = Select(t=2, s=w2566, f=0) -> (s? t:f=w2561:i32)
                n1616 = property on="SELECT LAB05-2" class="RadioBtnsControl (strict)"("DisabledEnum"=w2559) -> ()  [unwired: 2 in, 2 out]
                n1617 = property on="SELECT LAB05-1" class="RadioBtnsControl (strict)"("DisabledEnum"=w2560) -> ()  [unwired: 2 in, 2 out]
                n1618 = property on="SELECT LAB03-2" class="RadioBtnsControl (strict)"("DisabledEnum"=w2563) -> ()  [unwired: 2 in, 2 out]
                n1619 = property on="SELECT LAB04-1" class="RadioBtnsControl (strict)"("DisabledEnum"=w2562) -> ()  [unwired: 2 in, 2 out]
                n1620 = property on="SELECT LAB04-2" class="RadioBtnsControl (strict)"("DisabledEnum"=w2561) -> ()  [unwired: 2 in, 2 out]
                n1621 = property on="SET LAB05-2" class="Clust (strict)"("DisabledEnum"=w2559) -> ()  [unwired: 2 in, 2 out]
                n1622 = property on="SET LAB05-1" class="Clust (strict)"("DisabledEnum"=w2560) -> ()  [unwired: 2 in, 2 out]
                n1623 = property on="SET LAB03-2" class="Clust (strict)"("DisabledEnum"=w2563) -> ()  [unwired: 2 in, 2 out]
                n1624 = property on="SET LAB04-1" class="Clust (strict)"("DisabledEnum"=w2562) -> ()  [unwired: 2 in, 2 out]
                n1625 = property on="SET LAB04-2" class="Clust (strict)"("DisabledEnum"=w2561) -> ()  [unwired: 2 in, 2 out]
                n1626 = property on="O/I  LAB05-2" class="Bool (strict)"("DisabledEnum"=w2559) -> ()  [unwired: 2 in, 2 out]
                n1627 = property on="O/I  LAB05-1" class="Bool (strict)"("DisabledEnum"=w2560) -> ()  [unwired: 2 in, 2 out]
                n1628 = property on="O/I  LAB04-1" class="Bool (strict)"("DisabledEnum"=w2562) -> ()  [unwired: 2 in, 2 out]
